vi "FTW-CodeGen-Image.vi"(0 "State In":T1, 5 "XRef":refnum<vi>) -> (4 "Image":picture)   [LabVIEW 2013, in "FTW-SQLite-Fetch.xnode"]
uses:
  FTW-SQLite-Fetch.xnode
  FTW-CodeGen-State.ctl
panel:
  # "Inputs"
  # "Outputs"
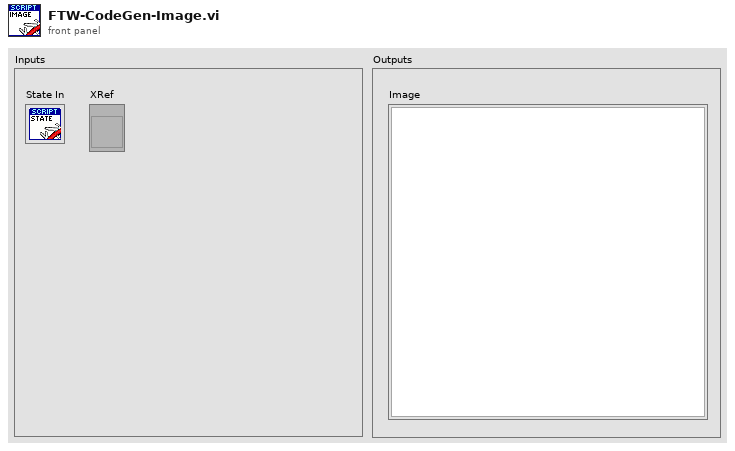
[diagram p1: front panel]
types:
  T1 = typedef "FTW-SQLite-Fetch.xnode/FTW-CodeGen-State.ctl" = cluster{"Dummy":string}
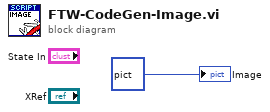
[diagram p0: block diagram]
diagram:
  "Image" <- picture bytes[3232] ("Picture")
